vi "Extrae_ScanField.vi"(10 "F string":string="Scan Field from 0.000Tesla to 0.500Tesla at 1.000Tesla/min, in 50 steps, Vuelta") -> (1 "Array F":string[](array[string]))   [LabVIEW 2017]
panel:
  out "Vuelta":bool
  out "Numeric":i32
  # "Set Magnetic Field 0.0Oe at 100.0Oe/sec, Linear, Persistent"
  # "Scan Field from 0.000Tesla to 0.500Tesla at 1.000Tesla/min, in 50 steps, Vuelta"
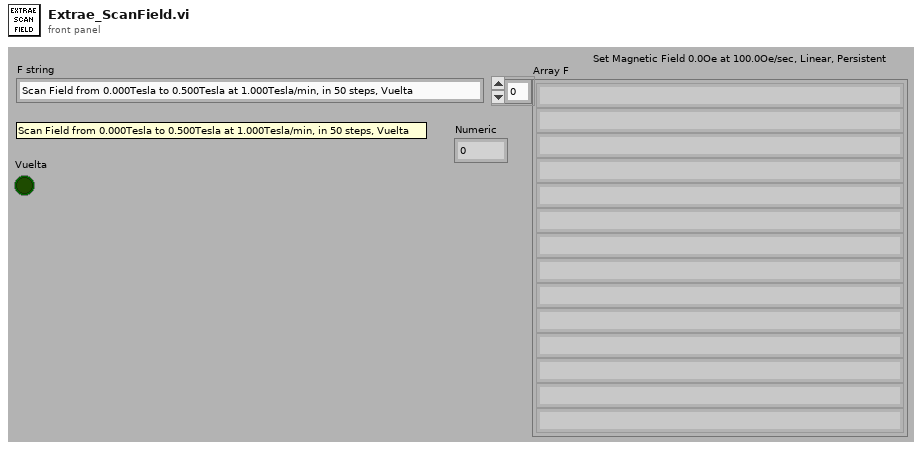
[diagram p1: front panel]
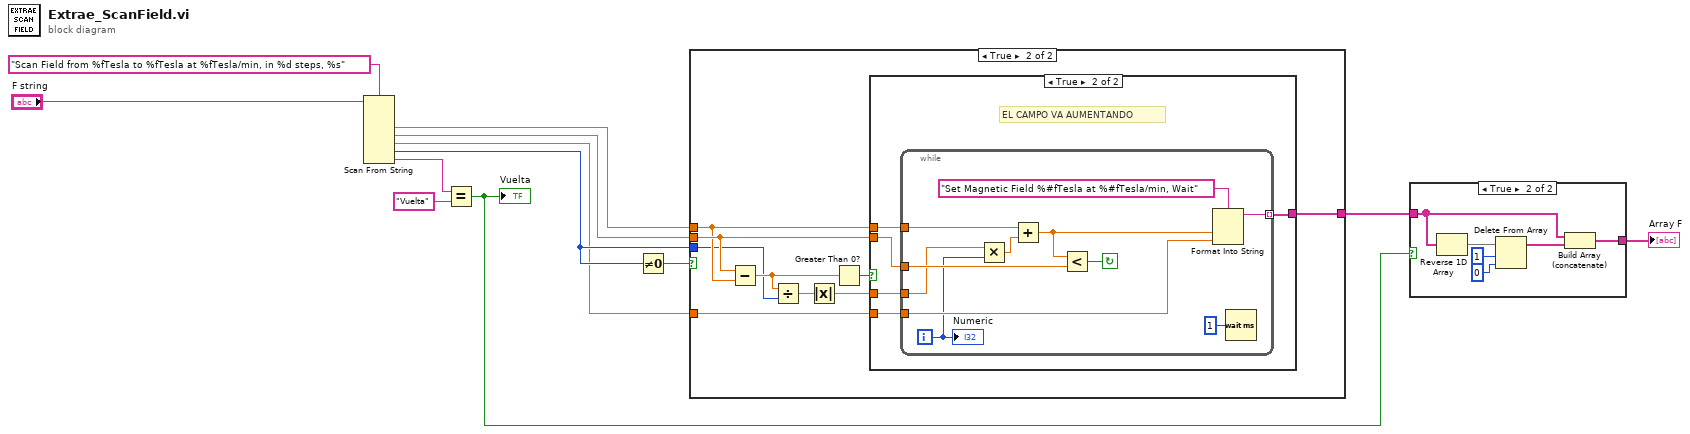
[diagram p0: block diagram]
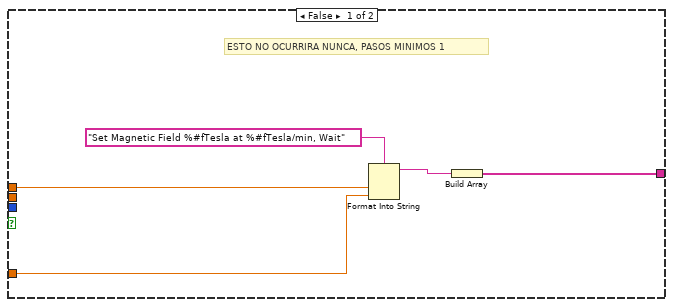
[diagram p3: hidden frame]
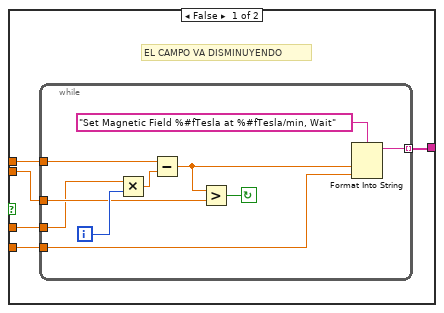
[diagram p4: hidden frame]
diagram:
  n1 = Scan From String(format string="Scan Field from %fTesla to %fTesla at %fTesla/min, in %d steps, %s", input string="F string") -> (output 1=w9:dbl, output 2=w8:dbl, output 3=w6:dbl, output 4=w7:i32, output 5=w5:string)  [unwired: 7 in, 3 out]
  n2 = Equal?(x=w5, y="Vuelta") -> (x = y?=w1:bool)
  "Vuelta" <- w1
  n3 = Not Equal To 0?(x=w7) -> (x != 0?=w10:bool)
  n4 = case shown="True" w10 {
    tunnel: w8 -> [_ w25]
    tunnel: w9 -> [w16 w24]
    tunnel: w7 -> [_ w20]
    tunnel: w6 -> [w15 w23]
    tunnel: [w13 w22] -> w3
    frame False {
      # "ESTO NO OCURRIRA NUNCA, PASOS MINIMOS 1"
      n5 = Format Into String(format string="Set Magnetic Field %#fTesla at %#fTesla/min, Wait", w16, w15) -> (resulting string=w14:string)  [unwired: 2 in, 1 out]
      n6 = Build Array(w14) -> (w13:string[])
    }
    frame True {
      n7 = Subtract(x=w25, y=w24) -> (x-y=w21:dbl)
      n8 = Divide(x=w21, y=w20) -> (x/y=w19:dbl)
      n9 = Absolute Value(x=w19) -> (abs(x)=w18:dbl)
      n10 = Greater Than 0?(x=w21) -> (x > 0?=w26:bool)
      n11 = case shown="True" w26 {
        tunnel: [w28 w43] -> w22
        tunnel: w25 -> [w31 w46]
        tunnel: w24 -> [w30 w45]
        tunnel: w23 -> [w29 w44]
        tunnel: w18 -> [w27 w42]
        frame False {
          # "EL CAMPO VA DISMINUYENDO"
          n12 = while {
            tunnel: w30 -> [w39]
            tunnel: w31 -> [w38]
            tunnel: w29 -> [w35]
            tunnel: [w33] -> w28 mode=indexing
            tunnel: w27 -> [w32]
            i -> [w41]
            stop <- w37 continue-if-true
            n13 = Multiply(x=w32, y=w41) -> (x*y=w40:dbl)
            n14 = Subtract(x=w39, y=w40) -> (x-y=w36:dbl)
            n15 = Greater?(x=w36, y=w38) -> (0:w37:bool)
            n16 = Format Into String(format string="Set Magnetic Field %#fTesla at %#fTesla/min, Wait", w36, w35) -> (resulting string=w33:string)  [unwired: 2 in, 1 out]
          }
        }
        frame True {
          # "EL CAMPO VA AUMENTANDO"
          n17 = while {
            tunnel: w45 -> [w57]
            tunnel: w46 -> [w56]
            tunnel: w44 -> [w53]
            tunnel: [w51] -> w43 mode=indexing
            tunnel: w42 -> [w48]
            i -> [w49]
            stop <- w55 continue-if-true
            n18 = Multiply(x=w48, y=w49) -> (x*y=w47:dbl)
            n19 = Add(x=w57, y=w47) -> (x+y=w54:dbl)
            n20 = Less?(x=w54, y=w56) -> (x < y?=w55:bool)
            n21 = Format Into String(format string="Set Magnetic Field %#fTesla at %#fTesla/min, Wait", w54, w53) -> (resulting string=w51:string)  [unwired: 2 in, 1 out]
            n22 = Wait (ms)(milliseconds to wait=u32 1) -> ()  [unwired: 1 out]
            "Numeric" <- w49
          }
        }
      }
    }
  }
  n23 = case shown="True" w1 {
    tunnel: w3 -> [w58 w59]
    tunnel: [w58 w60] -> w2
    frame False {
    }
    frame True {
      n24 = Reverse 1D Array(array=w59) -> (reversed array=w63:string[])
      n25 = Delete From Array(array=w63, length=1, index=0) -> (array with subset deleted=w61:string[])  [unwired: 1 out]
      n26 = Build Array (concatenate)(w59, w61) -> (w60:string[])
    }
  }
  "Array F" <- w2
